vi "Gated Counter.vi"() -> ()   [LabVIEW 2020]
uses:
  <vilib>/DAQmx/read.llb/DAQmx Read (Counter U32 1Chan 1Samp).vi
  <vilib>/DAQmx/create/channels.llb/DAQmx Create Channel (CI-Count Edges).vi
  <vilib>/DAQmx/create/channels.llb/DAQmx Create Channel (CO-Pulse Generation-Frequency).vi
  <vilib>/DAQmx/configure/timing.llb/DAQmx Timing (Implicit).vi
  <vilib>/DAQmx/create/channels.llb/DAQmx Create Channel (CO-Pulse Generation-Time).vi
  <vilib>/DAQmx/configure/trigger.llb/DAQmx Start Trigger (Digital Edge).vi
  <vilib>/DAQmx/miscellaneous.llb/DAQmx Fill In Error Info.vi
  <resource>/objmgr/daqmx.rc
panel:
  out "Counted Waves":u32
  in  "Reset Count":bool
  in  "stop":bool
  in  "Pulse Train Pin":tag
  in  "Gate Output":tag
  in  "Gate input":tag
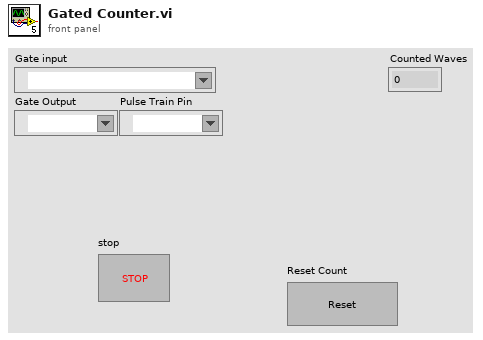
[diagram p1: front panel]
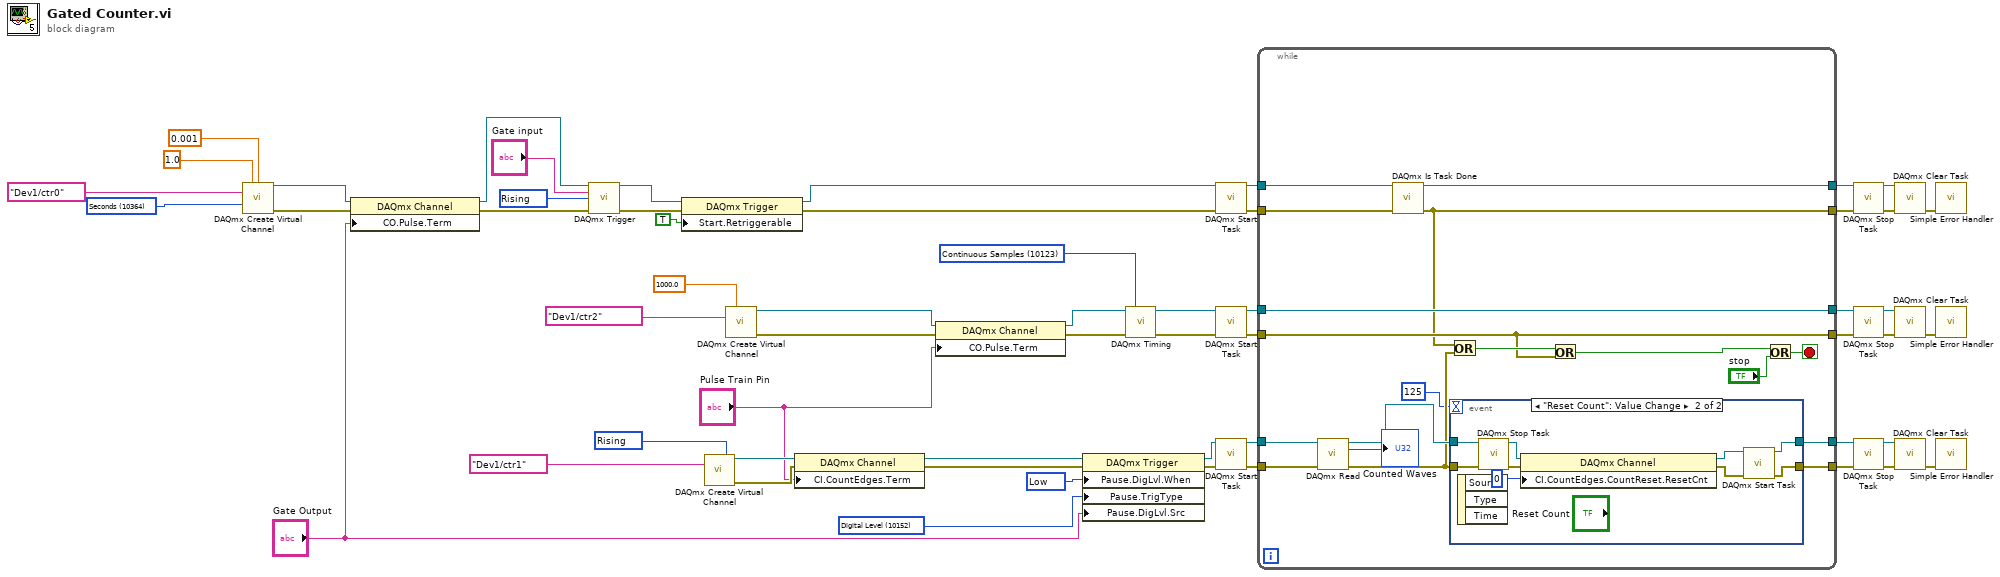
[diagram p0: block diagram]
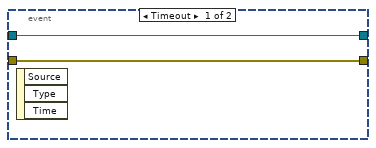
[diagram p2: hidden frame]
diagram:
  w32 = 10123 items=["Finite Samples"=10178, "Continuous Samples"=10123, "Hardware Timed Single Point"=12522] ("sample mode")
  w33 = 10364 items=["Seconds"=10364] ("units")
  w34 = 10214 items=["High"=10192, "Low"=10214] ("Pause.DigLvl.When")
  w35 = 10152 items=["Analog Level"=10101, "Analog Window"=10103, "Digital Level"=10152, "Digital Pattern"=10398, "None"=10230] ("Pause.TrigType")
  w42 = 10280 items=["Rising"=10280, "Falling"=10171] ("edge")
  w52 = 10280 items=["Rising"=10280, "Falling"=10171] ("edge")
  n1 = call-poly <vilib>:"DAQmx Create Virtual Channel.vi"("high time"=1.0, "low time"=0.001, "counter"=tag "Dev1/ctr0", "units"=w33) -> ("task out"=w49:refnum<k21>, "error out"=w48:errorcluster)  [unwired: 10 in]
  n2 = property class="DAQmx Channel"(reference=w49, error in=w48, "CO.Pulse.Term"="Gate Output") -> (reference out=w47:refnum<k21>, error out=w46:errorcluster)
  n3 = call-poly <vilib>:"DAQmx Trigger.vi"("task/channels in"=w47, "source"="Gate input", "edge"=w42, "error in"=w46) -> ("task out"=w57:refnum<k21>, "error out"=w56:errorcluster)  [unwired: 10 in]
  n4 = property class="DAQmx Trigger"(reference=w57, error in=w56, "Start.Retriggerable"=TRUE) -> (reference out=w4:refnum<k21>, error out=w3:errorcluster)
  n5 = call-poly <vilib>:"DAQmx Create Virtual Channel.vi"("edge"=w52, "counter"=tag "Dev1/ctr1") -> ("task out"=w51:refnum<k21>, "error out"=w50:errorcluster)  [unwired: 12 in]
  n6 = call-poly <vilib>:"DAQmx Create Virtual Channel.vi"("frequency"=1000.0, "counter"=tag "Dev1/ctr2") -> ("task out"=w41:refnum<k21>, "error out"=w40:errorcluster)  [unwired: 12 in]
  n7 = property class="DAQmx Channel"(reference=w51, error in=w50, "CI.CountEdges.Term"="Pulse Train Pin") -> (reference out=w38:refnum<k21>, error out=w37:errorcluster)
  n8 = property class="DAQmx Channel"(reference=w41, error in=w40, "CO.Pulse.Term"="Pulse Train Pin") -> (reference out=w31:refnum<k21>, error out=w30:errorcluster)
  n9 = property class="DAQmx Trigger"(reference=w38, error in=w37, "Pause.DigLvl.When"=w34, "Pause.TrigType"=w35, "Pause.DigLvl.Src"="Gate Output") -> (reference out=w6:refnum<k21>, error out=w5:errorcluster)
  n10 = call-poly <vilib>:"DAQmx Timing.vi"("task/channels in"=w31, "sample mode"=w32, "error in"=w30) -> ("task out"=w25:refnum<k21>, "error out"=w24:errorcluster)  [unwired: 11 in]
  n11 = call <vilib>:"DAQmx Start Task.vi"("task/channels in"=w4, "error in"=w3) -> ("task out"=w23:refnum<k21>, "error out"=w22:errorcluster)  [unwired: 12 in]
  n12 = call <vilib>:"DAQmx Start Task.vi"("task/channels in"=w25, "error in"=w24) -> ("task out"=w27:refnum<k21>, "error out"=w26:errorcluster)  [unwired: 12 in]
  n13 = call <vilib>:"DAQmx Start Task.vi"("task/channels in"=w6, "error in"=w5) -> ("task out"=w29:refnum<k21>, "error out"=w28:errorcluster)  [unwired: 12 in]
  n14 = while {
    tunnel: w29 -> [w69]
    tunnel: w28 -> [w68]
    tunnel: w27 -> [w71]
    tunnel: w26 -> [w70]
    tunnel: w23 -> [w67]
    tunnel: w22 -> [w66]
    tunnel: [w65] -> w11
    tunnel: [w64] -> w10
    tunnel: [w62] -> w9
    tunnel: [w71] -> w8
    tunnel: [w70] -> w7
    tunnel: [w60] -> w1
    stop <- w74 stop-if-true
    n15 = call-poly <vilib>:"DAQmx Read.vi"("task/channels in"=w69, "error in"=w68) -> ("task out"=w63:refnum<k21>, "data"=→"Counted Waves":u32, "error out"=w61:errorcluster)  [unwired: 11 in]
    n16 = call <vilib>:"DAQmx Is Task Done.vi"("task/channels in"=w67, "error in"=w66) -> ("task out"=w65:refnum<k21>, "error out"=w64:errorcluster)  [unwired: 11 in, 1 out]
    n17 = Or(x=w64, y=w61) -> (x .or. y?=w72:bool)
    n18 = event shown="[1] \"Reset Count\": Value Change" {
      selector: _ -> [_ _]
      dyn-events: _ -> [_ _]
      timeout: 125 -> [_ _]
      tunnel: w63 -> [w77 w85]
      tunnel: [w77 w79] -> w62
      tunnel: w61 -> [w76 w84]
      tunnel: [w76 w78] -> w60
      event Timeout {
        n19 = event-data() -> ()  [unwired: 1 in, 3 out]
      }
      event "Reset Count": Value Change {
        n20 = event-data() -> ()  [unwired: 1 in, 3 out]
        n21 = call <vilib>:"DAQmx Stop Task.vi"("task/channels in"=w85, "error in"=w84) -> ("task out"=w83:refnum<k21>, "error out"=w82:errorcluster)  [unwired: 12 in]
        n22 = property class="DAQmx Channel"(reference=w83, error in=w82, "CI.CountEdges.CountReset.ResetCnt"=u32 0) -> (reference out=w81:refnum<k21>, error out=w80:errorcluster)
        n23 = call <vilib>:"DAQmx Start Task.vi"("task/channels in"=w81, "error in"=w80) -> ("task out"=w79:refnum<k21>, "error out"=w78:errorcluster)  [unwired: 12 in]
      }
    }
    n24 = Or(x=w72, y=w70) -> (x .or. y?=w73:bool)
    n25 = Or(x=w73, y="stop") -> (x .or. y?=w74:bool)
  }
  n26 = call <vilib>:"DAQmx Stop Task.vi"("task/channels in"=w11, "error in"=w10) -> ("task out"=w17:refnum<k21>, "error out"=w16:errorcluster)  [unwired: 12 in]
  n27 = call <vilib>:"DAQmx Stop Task.vi"("task/channels in"=w8, "error in"=w7) -> ("task out"=w19:refnum<k21>, "error out"=w18:errorcluster)  [unwired: 12 in]
  n28 = call <vilib>:"DAQmx Stop Task.vi"("task/channels in"=w9, "error in"=w1) -> ("task out"=w21:refnum<k21>, "error out"=w20:errorcluster)  [unwired: 12 in]
  n29 = call <vilib>:"DAQmx Clear Task.vi"("task in"=w17, "error in"=w16) -> ("error out"=w13:errorcluster)  [unwired: 13 in]
  n30 = call <vilib>:"DAQmx Clear Task.vi"("task in"=w19, "error in"=w18) -> ("error out"=w15:errorcluster)  [unwired: 13 in]
  n31 = call <vilib>:"DAQmx Clear Task.vi"("task in"=w21, "error in"=w20) -> ("error out"=w14:errorcluster)  [unwired: 13 in]
  n32 = call <vilib>:"Simple Error Handler.vi"("error in (no error)"=w13) -> ()  [unwired: 4 in, 5 out]
  n33 = call <vilib>:"Simple Error Handler.vi"("error in (no error)"=w15) -> ()  [unwired: 4 in, 5 out]
  n34 = call <vilib>:"Simple Error Handler.vi"("error in (no error)"=w14) -> ()  [unwired: 4 in, 5 out]
